vi "VisitLVArrayType.vi"(8 "error in (no error)":errorcluster, 10 "LVArrayType":refnum<class "LVArrayType.lvclass">, 11 "NextGenXMLTypeGenerator in":refnum<class "NextGenXMLTypeGenerator.lvclass">) -> (0 "error out":errorcluster, 3 "NextGenXMLTypeGenerator out":refnum<class "NextGenXMLTypeGenerator.lvclass">)   [LabVIEW 2020, in "Web Service Description.lvlib" / "NextGenXMLTypeGenerator.lvclass"]
uses:
  <vilib>/AppBuilder/Engine/WebServiceDescription/NextGenXMLTypeGenerator/NextGenXMLTypeGenerator.lvclass
  e:/builds/penguin/labview/branches/2020/dev/dist/vi.lib/AppBuilder/Engine/WebServiceDescription/LVDataTypes/LVTypeVisitor/LVTypeVisitor.lvclass
  <vilib>/AppBuilder/Engine/WebServiceDescription/LVDataTypes/LVArrayType/LVArrayType.lvclass
  <vilib>/AppBuilder/Engine/WebServiceDescription/XMLGen/ValuePair.ctl
  <vilib>/AppBuilder/Engine/WebServiceDescription/NextGenXMLTypeGenerator/NextGenXMLTypeGenerator.lvclass/NextGenXMLTypeGenerator.ctl
  <vilib>/AppBuilder/Engine/WebServiceDescription/GetTypeAttributesVisitor/GetTypeAttributesVisitor.lvclass
  <vilib>/AppBuilder/Engine/WebServiceDescription/LVDataTypes/LVType/LVType.lvclass
  <vilib>/AppBuilder/Engine/WebServiceDescription/XMLGen/XMLGen.lvlib
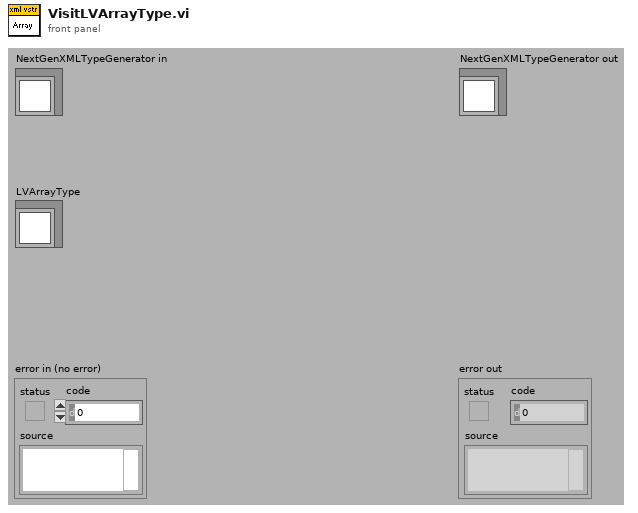
[diagram p1: front panel]
types:
  T1 = typedef "XMLGen.lvlib/ValuePair.ctl" = cluster{"Name":string, "Value":string}
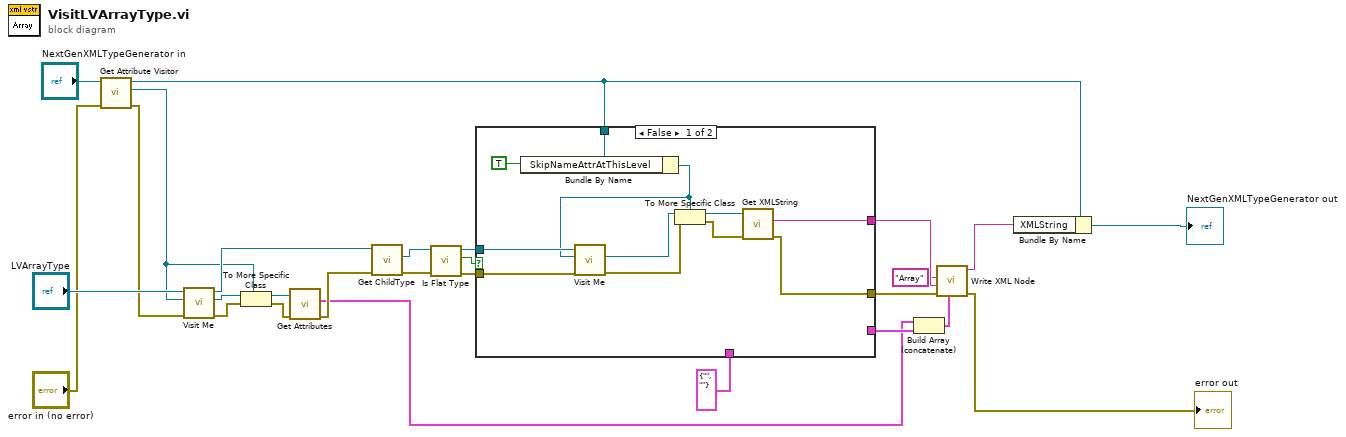
[diagram p0: block diagram]
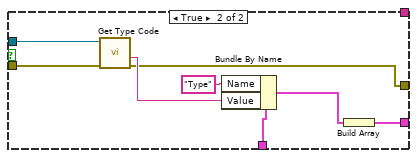
[diagram p2: hidden frame]
diagram:
  n1 = call <vilib>:"Get Attribute Visitor.vi"("error in (no error)"="error in (no error)", "NextGenXMLTypeGenerator in"="NextGenXMLTypeGenerator in") -> ("error out"=w2:errorcluster, "Attribute Visitor"=w1:refnum<class "GetTypeAttributesVisitor.lvclass">, "NextGenXMLTypeGenerator out"=w4:refnum<class "NextGenXMLTypeGenerator.lvclass">)  [unwired: 7 out]
  n2 = call-dynamic "Visit Me.vi"("error in (no error)"=w2, "Visitor In"=w1, "LVArrayType in"="LVArrayType") -> ("error out"=w12:errorcluster, "Visitor Out"=w13:refnum<class "LVTypeVisitor.lvclass">, "LVArrayType out"=w8:refnum<class "LVArrayType.lvclass">)  [unwired: 6 out]
  n3 = To More Specific Class(target class=w1, reference=w13, error in=w12) -> (specific class reference=w10:refnum<class "GetTypeAttributesVisitor.lvclass">, error out=w11:errorcluster)
  n4 = call <vilib>:"Get Attributes.vi"("error in (no error)"=w11, "GetTypeAttributesVisitor.lvclass in"=w10) -> ("error out"=w7:errorcluster, "Attributes"=w6:T1[])  [unwired: 8 out]
  n5 = call <vilib>:"Get ChildType.vi"("error in (no error)"=w7, "LVArrayType.lvclass in"=w8) -> ("error out"=w21:errorcluster, "ChildType"=w17:refnum<class "LVType.lvclass">)  [unwired: 8 out]
  n6 = call-dynamic "Is Flat Type.vi"("error in (no error)"=w21, "LVType in"=w17) -> ("error out"=w18:errorcluster, "Flat Type?"=w19:bool, "LVType out"=w16:refnum<class "LVType.lvclass">)  [unwired: 7 out]
  n7 = case shown="False" w19 {
    tunnel: [w38 w39] -> w26
    tunnel: [w37 _] -> w25
    tunnel: w4 -> [w30 _]
    tunnel: w18 -> [w32 w46]
    tunnel: w16 -> [w31 w45]
    tunnel: T1 {"Name"="", "Value"=""} ("Attribute") -> [_ w43]
    tunnel: [_ w40] -> w14
    frame False {
      n8 = Bundle By Name(cluster=w30, "SkipNameAttrAtThisLevel"=TRUE) -> (w28:refnum<class "NextGenXMLTypeGenerator.lvclass">)
      n9 = call-dynamic "Visit Me.vi"("error in (no error)"=w32, "Visitor In"=w28, "LVType in"=w31) -> ("error out"=w34:errorcluster, "Visitor Out"=w33:refnum<class "LVTypeVisitor.lvclass">)  [unwired: 7 out]
      n10 = To More Specific Class(target class=w28, reference=w33, error in=w34) -> (specific class reference=w35:refnum<class "NextGenXMLTypeGenerator.lvclass">, error out=w36:errorcluster)
      n11 = call <vilib>:"Get XMLString.vi"("error in (no error)"=w36, "NextGenXMLTypeGenerator.lvclass in"=w35) -> ("error out"=w38:errorcluster, "XMLString"=w37:string)  [unwired: 8 out]
    }
    frame True {
      n12 = call <vilib>:"Get Type Code.vi"("error in (no error)"=w46, "LVType.lvclass in"=w45) -> ("error out"=w39:errorcluster, "TypeCodeString"=w42:string)  [unwired: 8 out]
      n13 = Bundle By Name(cluster=w43, "Name"="Type", "Value"=w42) -> (w41:T1)
      n14 = Build Array(w41) -> (w40:T1[])
    }
  }
  n15 = Build Array (concatenate)(w6, w14) -> (w20:T1[])
  n16 = call <vilib>:"Write XML Node.vi"("attributes"=w20, "error in (no error)"=w26, "body"=w25, "node"="Array") -> ("error out"=→"error out":errorcluster, "resulting string"=w27:string)  [unwired: 1 in, 5 out]
  n17 = Bundle By Name(cluster=w4, "XMLString"=w27) -> (→"NextGenXMLTypeGenerator out":refnum<class "NextGenXMLTypeGenerator.lvclass">)
